vi "MH_SetInputChannelOffset.vi"(8 "error in (no error)":errorcluster, 9 "Offset":i32, 10 "channel":i32, 11 "devidx":i32) -> (0 "error out":errorcluster, 3 "return type":i32)   [LabVIEW 2019]
uses:
  <userlib>/MultiHarp150/MH_DllPath_global.vi
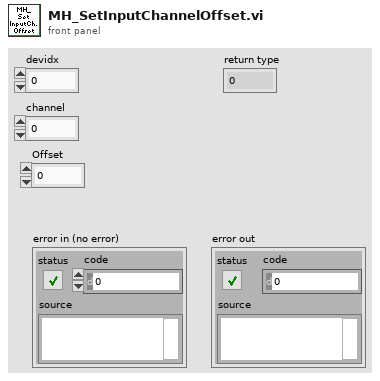
[diagram p1: front panel]
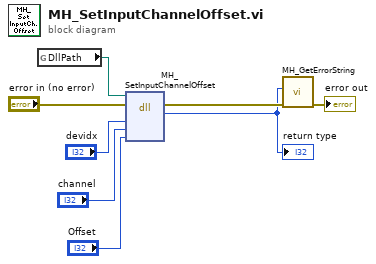
[diagram p0: block diagram]
diagram:
  n1 = global read "MH_DllPath_global.vi" "DllPath"() -> (w7:path)
  n2 = dll-call lib="MHLib64.dll" fn="MH_SetInputChannelOffset"(path in=w7, error in="error in (no error)", "devidx"="devidx", "channel"="channel", "Offset"="Offset") -> (error out=w5:errorcluster, "return type"=w4:i32)  [unwired: 4 in, 1 out]
  "return type" <- w4
  n3 = call <userlib>:"MH_GetErrorString.vi"("error in (no error)"=w5, "code"=w4) -> ("error out"=→"error out":errorcluster)  [unwired: 7 in, 2 out]
